vi "RunVI.vi"(2 "Numeric Input":dbl format="%.2f", 3 "Base":dbl format="%.2f", 4 "VI Refnum":refnum<vi>) -> (0 "error out":errorcluster, 1 "Numeric Output":dbl format="%.2f")   [LabVIEW 2011]
panel:
  in  "Ctl Refnum":refnum<vi>
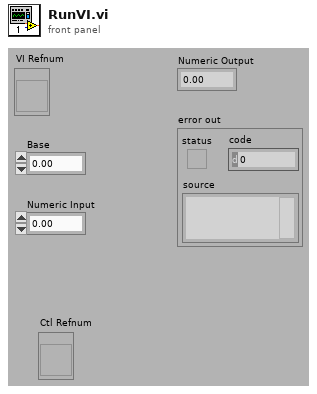
[diagram p1: front panel]
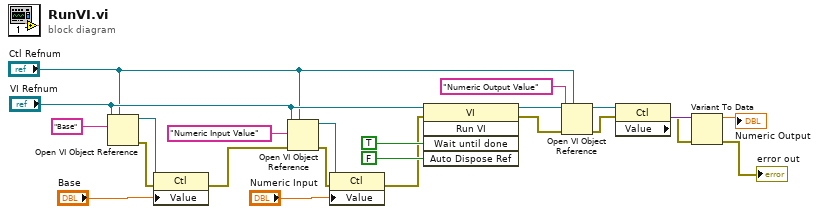
[diagram p0: block diagram]
diagram:
  n1 = Open VI Object Reference(7:"Ctl Refnum", 10:"Base" ("name/order"), 11:"VI Refnum") -> (0:w8:errorcluster, 3:w22:refnum<vi>)  [unwired: 1 in]
  n2 = property class="Ctl"(reference=w22, error in=w8, "Value"="Base") -> (error out=w7:errorcluster)  [unwired: 1 out]
  n3 = Open VI Object Reference(7:"Ctl Refnum", 8:w7, 10:"Numeric Input Value", 11:"VI Refnum") -> (0:w6:errorcluster, 3:w21:refnum<vi>)
  n4 = property class="Ctl"(reference=w21, error in=w6, "Value"="Numeric Input") -> (error out=w5:errorcluster)  [unwired: 1 out]
  n5 = invoke class="VI" method="Run VI"(reference="VI Refnum", error in=w5, "Wait until done"=TRUE, "Auto Dispose Ref"=FALSE) -> (reference out=w13:refnum<vi>, error out=w4:errorcluster)  [unwired: 1 in, 3 out]
  n6 = Open VI Object Reference(7:"Ctl Refnum", 8:w4, 10:"Numeric Output Value" ("name/order"), 11:w13) -> (0:w3:errorcluster, 3:w11:refnum<vi>)
  n7 = property class="Ctl"(reference=w11, error in=w3) -> (error out=w2:errorcluster, "Value"=w10:variant)  [unwired: 1 out]
  n8 = Variant To Data(error in=w2, Variant=w10) -> (data=→"Numeric Output":dbl, error out=→"error out":errorcluster)  [unwired: 1 in]
